vi "UpDateCalNewBfield.vi"(6 "2D in":T2, 9 "Camera Settings":T3, 10 "Cluster in":T1, 11 "B [T]":dbl) -> (2 "2D out":T2, 3 "Cluster out":T1)   [LabVIEW 2013]
uses:
  MagSpec_Bella/Controls/CameraSettings_File.ctl
  MagSpec_Bella/Controls/2D.ctl
  MagSpec_Bella/Controls/Calibration_Pixel_based.ctl
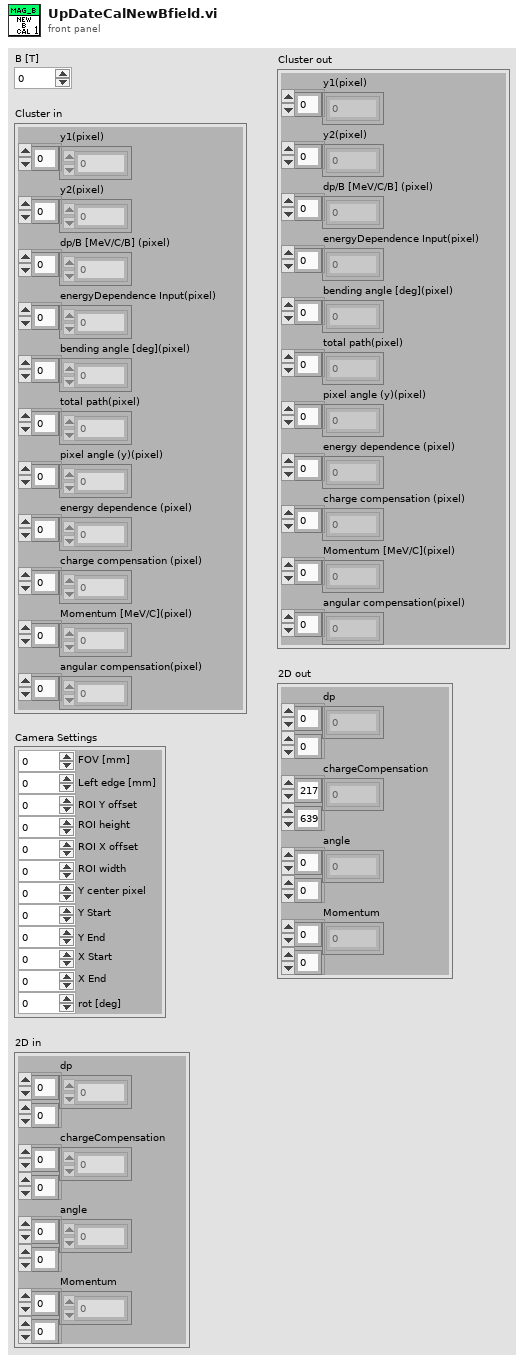
[diagram p1: front panel]
types:
  T1 = typedef "Calibration_Pixel_based.ctl" = cluster{"y1(pixel)":dbl[], "y2(pixel)":dbl[], "dp/B [MeV/C/B] (pixel)":dbl[], "energyDependence Input(pixel)":dbl[], "bending angle [deg](pixel)":dbl[], "total path(pixel)":dbl[], "pixel angle (y)(pixel)":dbl[], "energy dependence (pixel)":dbl[], "charge compensation (pixel)":dbl[], "Momentum [MeV/C](pixel)":dbl[], "angular compensation(pixel)":dbl[]}
  T2 = typedef "2D.ctl" = cluster{"dp":dbl[][], "chargeCompensation":dbl[][], "angle":dbl[][], "Momentum":dbl[][]}
  T3 = typedef "CameraSettings_File.ctl" = cluster{"FOV [mm]":dbl, "Left edge [mm]":dbl, "ROI Y offset":dbl, "ROI height":dbl, "ROI X offset":dbl, "ROI width":dbl, "Y center pixel":dbl, "Y Start":dbl, "Y End":dbl, "X Start":dbl, "X End":dbl, "rot [deg]":dbl}
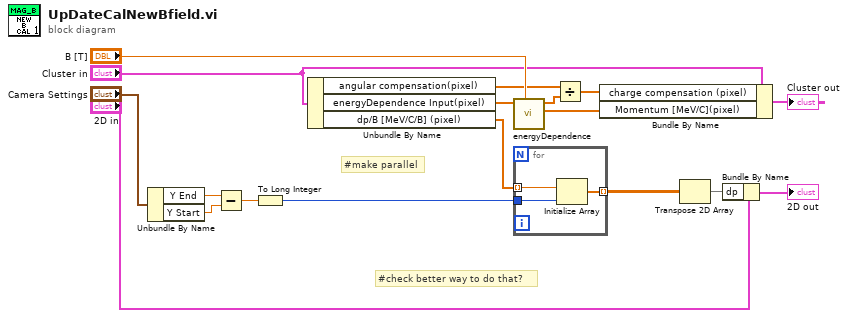
[diagram p0: block diagram]
diagram:
  # "#check better way to do that?"
  # "#make parallel"
  n1 = Unbundle By Name("Camera Settings") -> ("Y End"=w15:dbl, "Y Start"=w16:dbl)
  n2 = Subtract(x=w15, y=w16) -> (x-y=w17:dbl)
  n3 = To Long Integer(number=w17) -> (32bit integer=w12:i32)
  n4 = Unbundle By Name("Cluster in") -> ("angular compensation(pixel)"=w1:dbl[], "energyDependence Input(pixel)"=w2:dbl[], "dp/B [MeV/C/B] (pixel)"=w9:dbl[])
  n5 = call "energyDependence.vi"("B [T]"="B [T]", "energy Dep in"=w2) -> ("Momentum [MeV/C]"=w3:dbl[], "energy dependence"=w18:dbl[])  [unwired: 8 in]
  n6 = for {
    tunnel: w9 -> [w21] mode=indexing
    tunnel: [w20] -> w8 mode=indexing
    tunnel: w12 -> [w19]
    n7 = Initialize Array(w21, w19) -> (w20:dbl[])
  }
  n8 = Divide(x=w1, y=w18) -> (x/y=w14:dbl[])
  n9 = Bundle By Name(cluster="Cluster in", "charge compensation (pixel)"=w14, "Momentum [MeV/C](pixel)"=w3) -> (→"Cluster out":T1)
  n10 = Transpose 2D Array(2D array=w8) -> (transposed array=w13:dbl[][])
  n11 = Bundle By Name(cluster="2D in", "dp"=w13) -> (→"2D out":T2)
